vi "activate suction.vi"(8 "error in (no error)":errorcluster, 11 "Elevator Concrete in":refnum<class "Elevator Arm.lvclass">) -> (0 "error out":errorcluster, 3 "Elevator Concrete out":refnum<class "Elevator Arm.lvclass">)   [LabVIEW 2018, in "Elevator.lvlib" / "Elevator Arm.lvclass"]
doc: "It activates suction."
uses:
  Elevator Arm.lvclass
  <vilib>/Rock Robotics/WPI/ThirdParty/Phoenix-LabVIEW/Motor Controller/Controls/CTRE_Phoenix_MotorControl_ControlMode.ctl
  Elevator Arm.lvclass/Elevator Arm.ctl
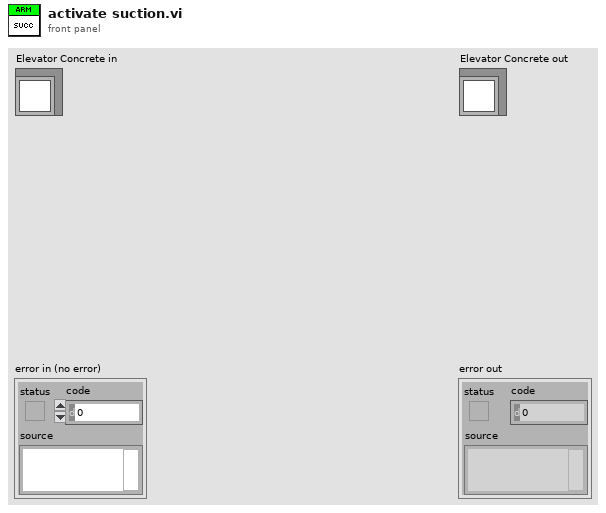
[diagram p1: front panel]
types:
  T1 = typedef "CTRE_Phoenix_MotorControl_ControlMode.ctl" = u16
  T2 = typedef "WPI_MotorControlDeviceRef.ctl" = cluster{"DeviceStatus":errorcluster, "Type":T3, "PWM":cluster{"PWM Channel":T4, "DeadBand":T5}, "CAN":cluster{"Device Number":u8, "SetOutput VI Ref":variant, "GetOutput VI Ref":variant, "Enable VI Ref":variant, "Disable VI Ref":variant, "Data":variant}, "Invert":bool, "DIO PWM":cluster{"PWM \"Enable\" Channel":T4, "DIOChannel":T6, "PWM Rate":dbl}}
  T3 = typedef "WPI_MotorControlType.ctl" = enum16{"PWM", "CAN", "DIO PWM"}
  T4 = typedef "FPGA_DIOPWMChannel.ctl" = enum8{"PWM 0", "PWM 1", "PWM 2", "PWM 3", "PWM 4", "PWM 5", "PWM 6", "PWM 7", "PWM 8", "PWM 9", "PWM MXP 0", "PWM MXP 1", "PWM MXP 2", "PWM MXP 3", "PWM MXP 4", "PWM MXP 5", "PWM MXP 6", "PWM MXP 7", "PWM MXP 8", "PWM MXP 9", "Invalid"}
  T5 = typedef "WPI_PWMDeadband.ctl" = cluster{"Name":string, "maxPositivePwm":i32, "minPositivePwm":i32, "centerPwm":i32, "maxNegativePwm":i32, "minNegativePwm":i32, "angularRange":u16}
  T6 = typedef "FPGA_DIOChannel.ctl" = enum8{"DIO 0", "DIO 1", "DIO 2", "DIO 3", "DIO 4", "DIO 5", "DIO 6", "DIO 7", "DIO 8", "DIO 9", "DIO MXP 0", "DIO MXP 1", "DIO MXP 2", "DIO MXP 3", "DIO MXP 4", "DIO MXP 5", "DIO MXP 6", "DIO MXP 7", "DIO MXP 8", "DIO MXP 9", "DIO MXP 10", "DIO MXP 11", "DIO MXP 12", "DIO MXP 13", "DIO MXP 14", "DIO MXP 15", "SPI Port CS1", "SPI Port CS2", "SPI Port CS3", "SPI Port MISO", "SPI Port MOSI", "Invalid"}
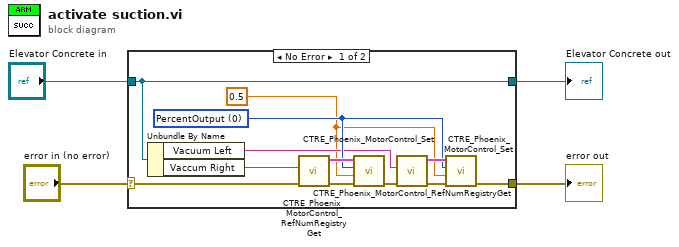
[diagram p0: block diagram]
diagram:
  n1 = case shown="No Error" "error in (no error)" {
    selector: "error in (no error)" -> [w8 w18]
    tunnel: [w14 w17] -> w2
    tunnel: "Elevator Concrete in" -> [w14 w17]
    tunnel: [w6 w18] -> w1
    frame No Error {
      w5 = 0.5
      w11 = T1 0 items=["PercentOutput"=0, "Position"=1, "Velocity"=2, "Current"=3, "Follower"=5, "MotionProfile"=6, "MotionMagic"=7, "MotionProfileArc"=10, "Disabled"=15] ("Control Mode")
      n2 = Unbundle By Name(w14) -> ("Vacuum Left"=w9:string, "Vaccum Right"=w10:string)
      n3 = call <vilib>:"CTRE_Phoenix_MotorControl_RefNumRegistryGet.vi"("error in (no error)"=w8, "refnum name"=w10) -> ("error out"=w16:errorcluster, "PhoenixMotorControlDevRef"=w15:T2)  [unwired: 8 in]
      n4 = call <vilib>:"CTRE_Phoenix_MotorControl_Set.vi"("error in (no error)"=w16, "Output"=w5, "Control Mode"=w11, "PhoenixMotorControlDevRef"=w15) -> ("error out"=w7:errorcluster)  [unwired: 6 in, 1 out]
      n5 = call <vilib>:"CTRE_Phoenix_MotorControl_RefNumRegistryGet.vi"("error in (no error)"=w7, "refnum name"=w9) -> ("error out"=w13:errorcluster, "PhoenixMotorControlDevRef"=w12:T2)  [unwired: 8 in]
      n6 = call <vilib>:"CTRE_Phoenix_MotorControl_Set.vi"("error in (no error)"=w13, "Output"=w5, "Control Mode"=w11, "PhoenixMotorControlDevRef"=w12) -> ("error out"=w6:errorcluster)  [unwired: 6 in, 1 out]
    }
    frame Error {
    }
  }
  "error out" <- w1
  "Elevator Concrete out" <- w2
